vi "Hello World.vi"   [LabVIEW 2018]
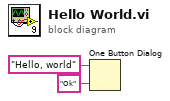
[diagram p0: block diagram]
diagram:
  n1 = One Button Dialog(message="Hello, world", button name ("OK")="Ok") -> ()  [unwired: 1 out]
